vi "RetrieveMetadataLiveOrPost.vi"(11 "ChannelsToGet":string[](array[string])) -> (3 "ChannelValues":dbl[](array[numeric]))   [LabVIEW 2021]
doc: "Given the Time Data Was Acquired (from MeasGlobal) in Take New Data mode, or Raw Data file (from MeasGlobal) in Post Process mode, this VI retrieves single values of the requested ADAM channels for the current measurement."
uses:
  Anemometry/Anemometry Sub Vis/Globals/Meas_global.vi
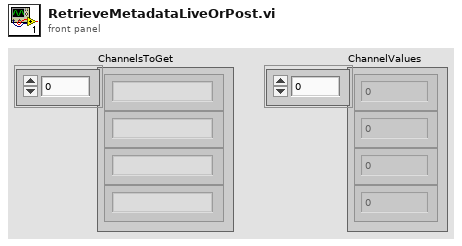
[diagram p1: front panel]
types:
  T1 = typedef "Post_Process.ctl" = enum16{"Take New Data", "Post Process Raw Data File"}
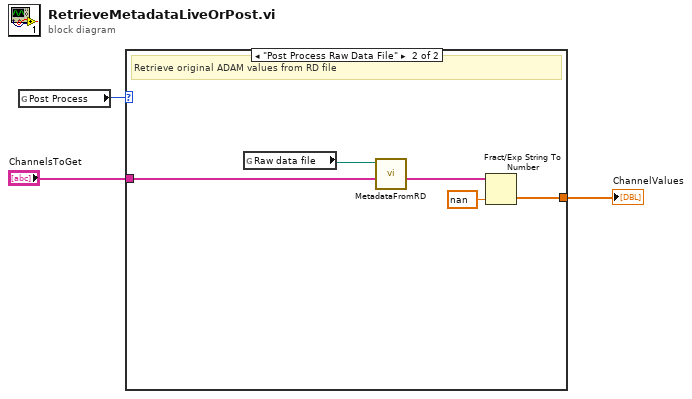
[diagram p0: block diagram]
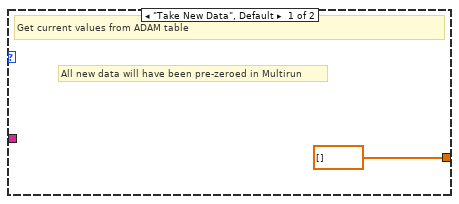
[diagram p2: hidden frame]
diagram:
  n1 = global read "Meas_global.vi" "Post Process"() -> (w2:T1)
  n2 = case shown="\"Post Process Raw Data File\"" w2 {
    tunnel: "ChannelsToGet" -> [_ w8]
    tunnel: [dbl[] [] w6] -> w3
    frame "Take New Data", Default {
      # "All new data will have been pre-zeroed in Multirun"
      # "Get current values from ADAM table"
    }
    frame "Post Process Raw Data File" {
      (unwired) string[] []
      # "Retrieve original ADAM values from RD file"
      n3 = global read "Meas_global.vi" "Raw data file"() -> (w9:path)
      n4 = call "MetadataFromRD.vi"("ChannelNames"=w8, "Raw data file"=w9) -> ("ValueStrings"=w7:string[])  [unwired: 8 in, 1 out]
      n5 = Fract/Exp String To Number(string=w7, default (0 dbl)=nan ("default (0 DBL)")) -> (number=w6:dbl[])  [unwired: 2 in, 1 out]
    }
  }
  "ChannelValues" <- w3
